vi "HLR_Mean NT.vi"(11 "Input":dbl[](array[numeric])=[1.0, 2.0, 3.0, 7.0]) -> (3 "Mean Data":dbl[](array[numeric]))   [LabVIEW 2025]
uses:
  <vilib>/ptbypt/NI_PtbyPt.lvlib
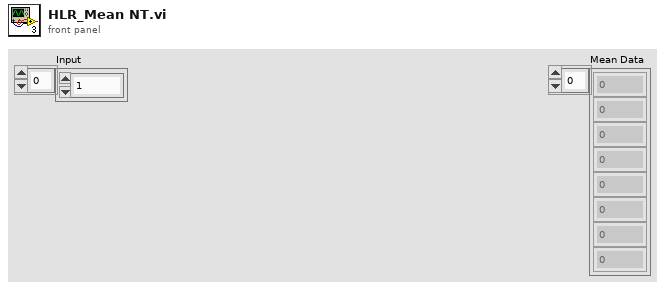
[diagram p1: front panel]
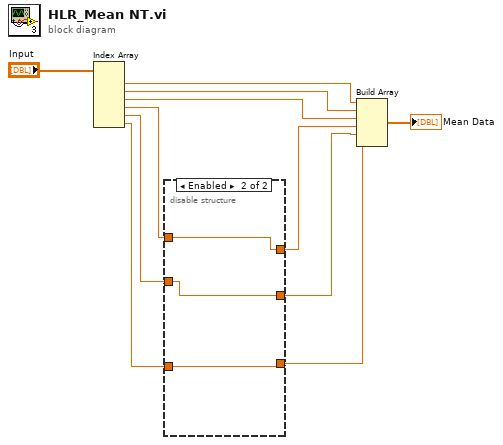
[diagram p0: block diagram]
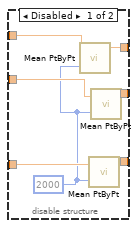
[diagram p2: hidden frame]
diagram:
  n1 = Index Array(array="Input") -> (element #1=w5:dbl, element #2=w4:dbl, element #3=w3:dbl, element #4=w10:dbl, element #5=w9:dbl, element #6=w2:dbl)  [unwired: 6 in]
  n2 = disable-structure shown="Enabled" {
    disable-tunnel: w10 -> [w18 w21]
    disable-tunnel: w9 -> [w17 w20]
    disable-tunnel: [w16 w21] -> w8
    disable-tunnel: [w15 w20] -> w7
    disable-tunnel: w2 -> [w14 w19]
    disable-tunnel: [w13 w19] -> w1
    frame Disabled {
      w12 = 2000 ("sample length")
      n3 = call <vilib>:"Mean PtByPt.vi"("x"=w18, "sample length"=w12) -> ("mean"=w16:dbl)  [unwired: 2 in, 1 out]
      n4 = call <vilib>:"Mean PtByPt.vi"("x"=w14, "sample length"=w12) -> ("mean"=w13:dbl)  [unwired: 2 in, 1 out]
      n5 = call <vilib>:"Mean PtByPt.vi"("x"=w17, "sample length"=w12) -> ("mean"=w15:dbl)  [unwired: 2 in, 1 out]
    }
    frame Enabled {
    }
  }
  n6 = Build Array(w5, w4, w3, w8, w7, w1) -> (→"Mean Data":dbl[])
